vi "exercise6.vi"() -> ()   [LabVIEW 2020]
uses:
  <vilib>/Analysis/NI_AALBase.lvlib
panel:
  in  "stop":bool
  in  "Plot Color":u32(colorbox)
  in  "Amplitude":dbl(knob) scale=0.0..10.0
  out "Waveform Chart":dbl[](graph)
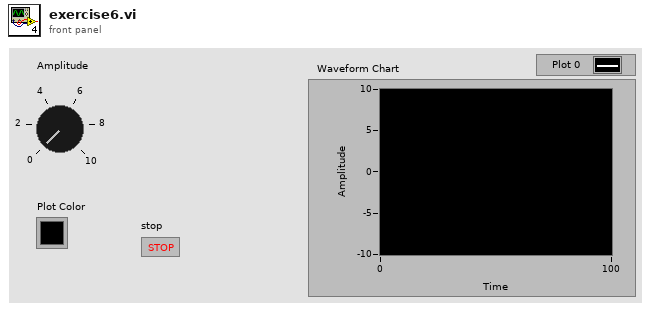
[diagram p1: front panel]
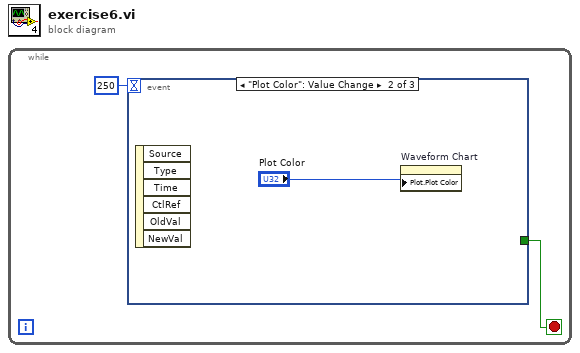
[diagram p0: block diagram]
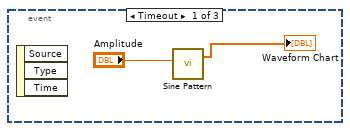
[diagram p2: hidden frame]
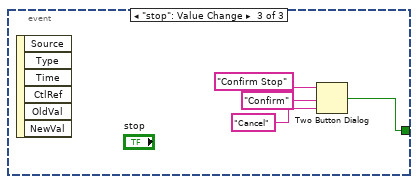
[diagram p3: hidden frame]
diagram:
  n1 = while {
    stop <- w2 stop-if-true
    n2 = event shown="[1] \"Plot Color\": Value Change" {
      selector: _ -> [_ _ _]
      dyn-events: _ -> [_ _ _]
      timeout: 250 -> [_ _ _]
      tunnel: [_ _ w6] -> w2
      event Timeout {
        n3 = event-data() -> ()  [unwired: 1 in, 3 out]
        n4 = call <vilib>:"Sine Pattern.vi"("amplitude"="Amplitude") -> ("Sinusoidal Pattern"=→"Waveform Chart":dbl[])  [unwired: 3 in, 1 out]
      }
      event "Plot Color": Value Change {
        n5 = event-data() -> ()  [unwired: 1 in, 6 out]
        n6 = property on="Waveform Chart" class="WFChart (strict)"("Plot.Plot Color"="Plot Color") -> ()  [unwired: 2 in, 2 out]
      }
      event "stop": Value Change {
        n7 = event-data() -> ()  [unwired: 1 in, 6 out]
        n8 = Two Button Dialog(message="Confirm Stop", 1:"Cancel" ("F button name (\"Cancel\")"), 2:"Confirm" ("T button name (\"OK\")")) -> (T button?=w6:bool)
      }
    }
  }
